vi "ELVIS R meas.vi"(0 "Device Name in":tag="Dev1", 2 "close session":bool, 11 "error in":errorcluster, 12 "Meas type":T1(ring)=enum."Resistance", 13 "Resistance Range (Ohms)":sgl(ring)=100000.0 items=["100ohm"=100, "1Kohm"=1000, "10Kohm"=10000, "100Kohm"=100000, "1Mohm"=1000000, "100Mohm"=1e+08]) -> (4 "Device Name out":tag="Dev1", 8 "Resistance (ohm)":dbl=12101.131778276253, 14 "Overrange":u16(ring) items=["In Range", "+Over", "-Over", "±Over"], 15 "error out":errorcluster)   [LabVIEW 2016]
doc: "Basic Digital Multimeter of NI ELVIS II configured to measure resistance\n\n\nPaul K Dixon\nP350\nCSUSB Physics"
uses:
  <vilib>/express/NI ELVISmx/misc.llb/ctl_ProductType.ctl
  <vilib>/DAQmx/read.llb/DAQmx Read (Analog 1D Wfm NChan NSamp).vi
  <vilib>/DAQmx/read.llb/DAQmx Read (Analog DBL 1Chan 1Samp).vi
  <vilib>/DAQmx/create/channels.llb/DAQmx Create Channel (AI-Voltage-Basic).vi
  <vilib>/DAQmx/create/channels.llb/DAQmx Create Channel (AI-Voltage-RMS).vi
  <vilib>/DAQmx/create/channels.llb/DAQmx Create Channel (AI-Current-Basic).vi
  <vilib>/DAQmx/create/channels.llb/DAQmx Create Channel (AI-Current-RMS).vi
  <vilib>/DAQmx/create/channels.llb/DAQmx Create Channel (AI-Resistance).vi
  <vilib>/DAQmx/create/channels.llb/DAQmx Create Channel (AO-FuncGen).vi
  <vilib>/DAQmx/configure/timing.llb/DAQmx Timing (Sample Clock).vi
  <vilib>/DAQmx/miscellaneous.llb/DAQmx Fill In Error Info.vi
  <vilib>/measure/matone.llb/Extract Single Tone Information 1 Chan.vi
  <resource>/objmgr/daqmx.rc
  <vilib>/measure/NI_MAPro.lvlib
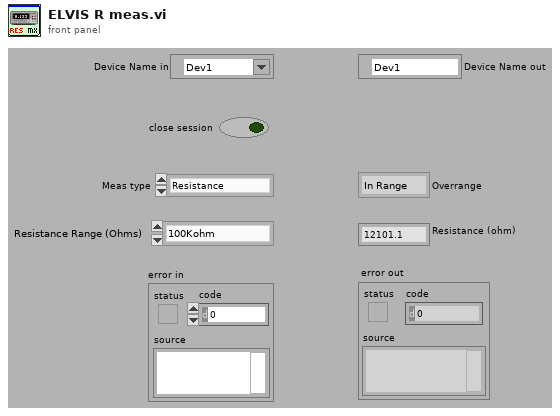
[diagram p1: front panel]
types:
  T1 = enum16{"Volts DC", "Volts AC", "Current DC", "Current AC", "Resistance", "Capacitance", "Inductance", "Diode", "Continuity", "Impedance"}
  T2 = typedef "ctl_ProductType.ctl" = enum16{"NI myDAQ", "NI ELVIS II", "NI ELVIS II+"}
  T3 = cluster{"approx freq. (optional)":dbl, "search (+/- % of Fsampl.)":dbl}
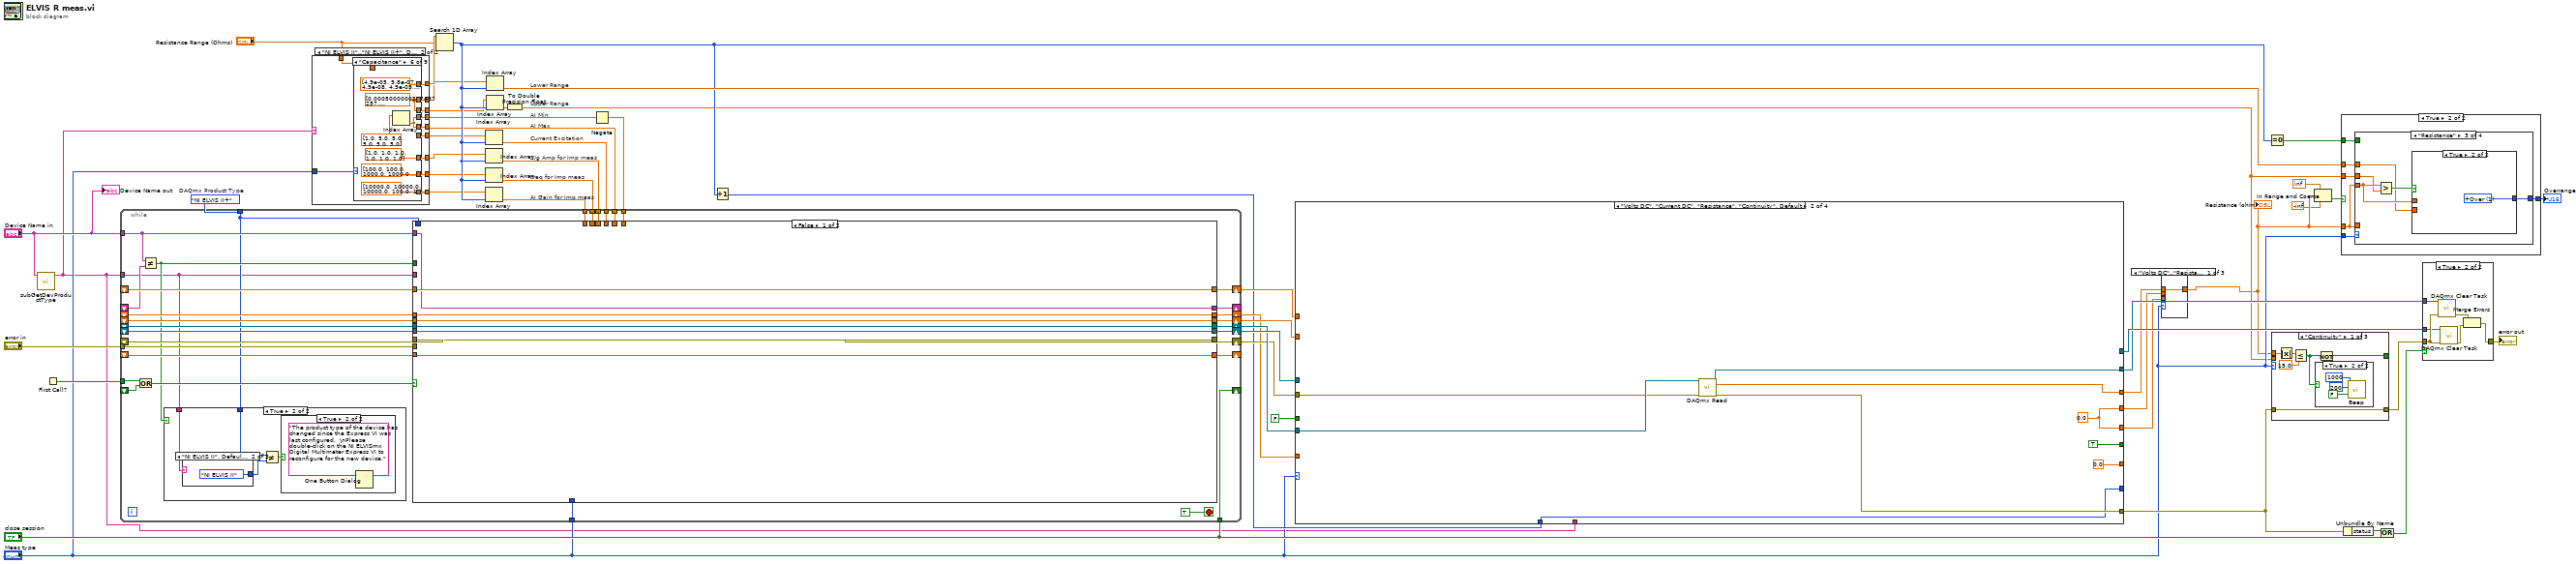
[diagram p0: block diagram]
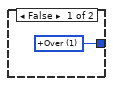
[diagram p2: hidden frame]
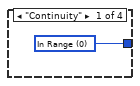
[diagram p3: hidden frame]
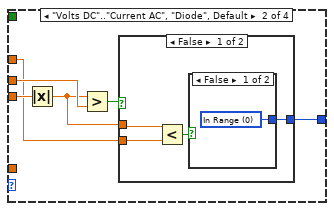
[diagram p4: hidden frame]
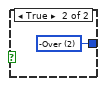
[diagram p5: hidden frame]
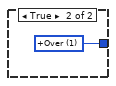
[diagram p6: hidden frame]
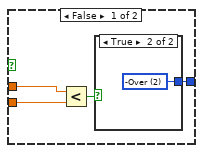
[diagram p7: hidden frame]
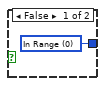
[diagram p8: hidden frame]
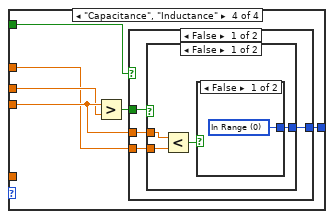
[diagram p9: hidden frame]
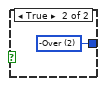
[diagram p10: hidden frame]
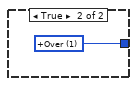
[diagram p11: hidden frame]
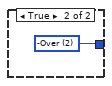
[diagram p12: hidden frame]
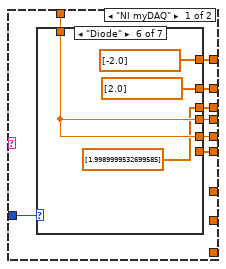
[diagram p13: hidden frame]
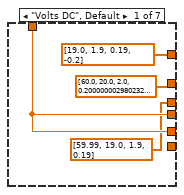
[diagram p14: hidden frame]
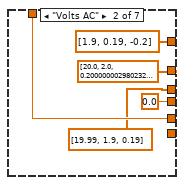
[diagram p15: hidden frame]
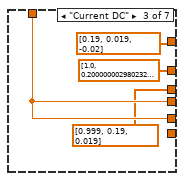
[diagram p16: hidden frame]
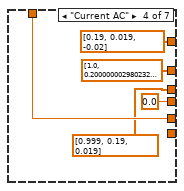
[diagram p17: hidden frame]
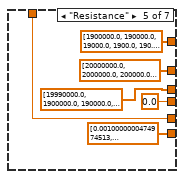
[diagram p18: hidden frame]
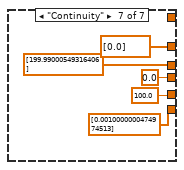
[diagram p19: hidden frame]
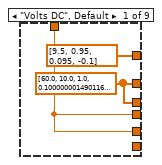
[diagram p20: hidden frame]
diagram:
  w7 = ctl_ProductType."NI ELVIS II+"  # DAQmx Product Type
  # "AI Max"
  # "Lower Range"
  # "Upper Range"
  # "AI Gain for Imp meas"
  # "Freq for Imp meas"
  # "S/g Amp for Imp meas"
  # "AI Min"
  # "Current Excitation"
  n1 = call <vilib>:"subGetDevProductType.vi"("activeDevice"="Device Name in") -> ("DevProductTypeValue"=w5:string)  [unwired: 9 in, 1 out]
  n2 = First Call?() -> (First Call?: T/F=w45:bool)
  n3 = case shown="\"NI ELVIS II\"..\"NI ELVIS II+\", Default" w5 {
    tunnel: [w58 w102] -> w20
    tunnel: [w57 w101] -> w19
    tunnel: [w52 w100] -> w18
    tunnel: [_ w99] -> w17
    tunnel: [_ w98] -> w15
    tunnel: [_ w97] -> w16
    tunnel: "Meas type" -> [w56 w96]
    tunnel: "Resistance Range (Ohms)" -> [w54 w95]
    tunnel: [w55 w94] -> w9
    tunnel: [w53 w93] -> w10
    tunnel: [w51 w92] -> w6
    frame "NI myDAQ" {
      n4 = case shown="\"Diode\"" w56 {
        tunnel: [dbl[] [19.0, 1.9, 0.19, -0.2] dbl[] [1.9, 0.19, -0.2] dbl[] [0.19, 0.019, -0.02] dbl[] [0.19, 0.019, -0.02] dbl[] [1900000.0, 190000.0, 19000.0, 1900.0, 190.0, -1000000000.0] sgl[] [-2.0] _] -> w58
        tunnel: [sgl[] [60.0, 20.0, 2.0, 0.2] sgl[] [20.0, 2.0, 0.2] sgl[] [1.0, 0.2, 0.02] sgl[] [1.0, 0.2, 0.02] sgl[] [20000000.0, 2000000.0, 200000.0, 20000.0, 2000.0, 200.0] sgl[] [2.0] sgl[] [0.0]] -> w57
        tunnel: [w60 sgl 0.0 ("Continuity Input Limits (Ohms)") w69 sgl 0.0 ("Continuity Input Limits (Ohms)") sgl 0.0 ("Continuity Input Limits (Ohms)") w86 sgl 0.0 ("Continuity Input Limits (Ohms)")] -> w55
        tunnel: w54 -> [w60 w64 w69 w73 w79 w86 _]
        tunnel: [w60 w64 w69 w73 w79 w86 sgl 100.0 ("Continuity Input Limits (Ohms)")] -> w53
        tunnel: [_ _ _ _ sgl[] [0.001, 0.001, 0.001, 0.001, 0.001, 0.001] _ sgl[] [0.001]] -> w52
        tunnel: [dbl[] [59.99, 19.0, 1.9, 0.19] dbl[] [19.99, 1.9, 0.19] dbl[] [0.999, 0.19, 0.019] dbl[] [0.999, 0.19, 0.019] dbl[] [19990000.0, 1900000.0, 190000.0, 19000.0, 1900.0, 190.0] dbl[] [1.9989999532699585] dbl[] [199.99000549316406]] -> w51
        frame "Volts DC", Default {
        }
        frame "Volts AC" {
        }
        frame "Current DC" {
        }
        frame "Current AC" {
        }
        frame "Resistance" {
        }
        frame "Diode" {
        }
        frame "Continuity" {
        }
      }
    }
    frame "NI ELVIS II".."NI ELVIS II+", Default {
      n5 = case shown="\"Capacitance\"" w96 {
        tunnel: [dbl[] [9.5, 0.95, 0.095, -0.1] dbl[] [1.9, 0.19, -0.2] dbl[] [0.0] dbl[] [0.48, -0.5] dbl[] [900000.0, 99000.0, 9000.0, 900.0, 90.0, -1000000000.0] dbl[] [4.9e-05, 9.8e-07, 4.9e-08, 4.9e-09, 4.5e-10, inf] dbl[] [0.01, 0.001, 0.0001] dbl[] [0.95, 0.0] _] -> w102
        tunnel: [w103 w106 w110 w113 w117 w122 w129 w136 w139] -> w101
        tunnel: [_ _ _ _ sgl[] [5e-07, 5e-06, 1e-05, 0.0001, 0.001, 0.001] _ _ _ dbl[] [0.001]] -> w100
        tunnel: [_ _ _ _ _ dbl[] [1.0, 1.0, 1.0, 1.0, 1.0, 1.0] dbl[] [1.0, 0.5, 0.5] _ _] -> w99
        tunnel: [_ _ _ _ _ dbl[] [100.0, 100.0, 1000.0, 1000.0, 1000.0, 10000.0] dbl[] [1000.0, 1000.0, 10000.0] _ _] -> w98
        tunnel: [_ _ _ _ _ dbl[] [10000.0, 10000.0, 10000.0, 100.0, 1.0, 1.0] dbl[] [10000.0, 10000.0, 10000.0] _ _] -> w97
        tunnel: w95 -> [w104 w108 w111 w115 w119 _ _ w137 _]
        tunnel: [w104 sgl 0.0 ("Continuity Input Limits (Ohms)") w111 sgl 0.0 ("Continuity Input Limits (Ohms)") sgl 0.0 ("Continuity Input Limits (Ohms)") w123 w130 w137 0.0 ("Continuity Input Limits (Ohms)")] -> w94
        tunnel: [w104 w108 w111 w115 w119 w123 w130 w137 100.0 ("Continuity Input Limits (Ohms)")] -> w93
        tunnel: [w103 w106 w110 w113 w117 w122 w129 w136 w139] -> w92
        frame "Volts DC", Default {
          w103 = sgl[] [60.0, 10.0, 1.0, 0.1]
        }
        frame "Volts AC" {
          w106 = sgl[] [20.0, 2.0, 0.2]
        }
        frame "Current DC" {
          w110 = sgl[] [2.0]
        }
        frame "Current AC" {
          w113 = sgl[] [2.0, 0.5]
        }
        frame "Resistance" {
          w117 = sgl[] [100000000.0, 1000000.0, 100000.0, 10000.0, 1000.0, 100.0]
        }
        frame "Capacitance" {
          w122 = sgl[] [0.0005, 5e-05, 1e-06, 5e-08, 5e-09, 5e-10]
          n6 = Index Array(array=dbl[] [1.0, 5.0, 5.0, 5.0, 5.0, 5.0]) -> (element=w123:dbl)  [unwired: 1 in]
        }
        frame "Inductance" {
          w129 = sgl[] [0.1, 0.01, 0.001]
          n7 = Index Array(array=dbl[] [1.0, 1.0, 1.0]) -> (element=w130:dbl)  [unwired: 1 in]
        }
        frame "Diode" {
          w136 = sgl[] [10.0, 1.0]
        }
        frame "Continuity" {
          w139 = sgl[] [0.0]
        }
      }
    }
  }
  n8 = Search 1D Array(1D array=w19, element="Resistance Range (Ohms)") -> (index of element=w22:i32)  [unwired: 1 in]
  n9 = Index Array(array=w18, index=w22) -> (element=w39:dbl)
  n10 = Index Array(array=w17, index=w22) -> (element=w38:dbl)
  n11 = Index Array(array=w15, index=w22) -> (element=w37:dbl)
  n12 = Index Array(array=w16, index=w22) -> (element=w36:dbl)
  n13 = Index Array(array=w6, index=w22) -> (element=w40:dbl)
  n14 = Index Array(array=w20, index=w22) -> (element=w41:dbl)
  n15 = To Double Precision Float(number=w40) -> (double precision float=w11:dbl)
  n16 = Negate(x=w9) -> (-x=w8:dbl)
  n17 = while {
    tunnel: "error in" -> [w175]
    shift-right: [w174] -> w33
    shift-left: _ -> [w172]
    shift-right: [w170] -> _
    shift-left: _ -> [w169]
    tunnel: "close session" -> [w170]
    tunnel: w45 -> [w167]
    shift-right: [w173] -> w32
    shift-left: _ -> [w166]
    tunnel: "Meas type" -> [w165]
    shift-right: [w164] -> w34
    shift-left: _ -> [w163]
    shift-right: [w162] -> _
    shift-left: _ -> [w146]
    shift-right: [w161] -> w30
    shift-left: _ -> [w160]
    shift-right: [w159] -> _
    shift-left: _ -> [w158]
    shift-right: [w157] -> w31
    shift-left: _ -> [w156]
    shift-right: [w155] -> w35
    shift-left: _ -> [w154]
    tunnel: w5 -> [w143]
    tunnel: w39 -> [w151]
    tunnel: w10 -> [w152]
    tunnel: w38 -> [w150]
    tunnel: w37 -> [w149]
    tunnel: w36 -> [w153]
    tunnel: "Device Name in" -> [w147]
    tunnel: w8 -> [w148]
    tunnel: w7 -> [w144]
    stop <- TRUE stop-if-true
    n18 = Or(x=w167, y=w169) -> (x .or. y?=w168:bool)
    n19 = Not Equal?(x=w147, y=w146) -> (x != y?=w145:bool)
    n20 = case shown="True" w145 {
      tunnel: w144 -> [_ w178]
      tunnel: w143 -> [_ w176]
      frame False {
      }
      frame True {
        n21 = case shown="\"NI ELVIS II\", Default" w176 {
          tunnel: [ctl_ProductType."NI ELVIS II+" ("Product Type") ctl_ProductType."NI ELVIS II" ("Product Type") ctl_ProductType."NI myDAQ" ("Product Type")] -> w179
          frame "NI ELVIS II+" {
          }
          frame "NI ELVIS II", Default {
          }
          frame "NI myDAQ" {
          }
        }
        n22 = Not Equal?(x=w178, y=w179) -> (x != y?=w177:bool)
        n23 = case shown="True" w177 {
          frame False {
          }
          frame True {
            n24 = One Button Dialog(message="The product type of the device has changed since the Express VI was last configured.  \nPlease double-click on the NI ELVISmx Digital Multimeter Express VI to reconfigure for the new device.") -> ()  [unwired: 1 in, 1 out]
          }
        }
      }
    }
    n25 = case shown="False" w168 {
      tunnel: w175 -> [_ w213]
      tunnel: [w191 w199] -> w174
      tunnel: [w190 w197] -> w173
      tunnel: w172 -> [w191 _]
      tunnel: w166 -> [w190 _]
      tunnel: w165 -> [_ w206]
      tunnel: [w189 w198] -> w164
      tunnel: w163 -> [w189 _]
      tunnel: [w184 w195] -> w162
      tunnel: [w188 w196] -> w161
      tunnel: w160 -> [w188 _]
      tunnel: [w186 w205] -> w159
      tunnel: w158 -> [w186 w210]
      tunnel: [w187 w201] -> w157
      tunnel: w156 -> [w187 _]
      tunnel: [w185 w200] -> w155
      tunnel: w154 -> [w185 _]
      tunnel: w143 -> [_ w193]
      tunnel: w153 -> [_ w196]
      tunnel: w152 -> [_ w209]
      tunnel: w151 -> [_ w208]
      tunnel: w150 -> [_ w207]
      tunnel: w149 -> [_ w200]
      tunnel: w147 -> [w184 w195]
      tunnel: w148 -> [_ w194]
      tunnel: w144 -> [_ _]
      tunnel: w145 -> [_ w192]
      frame False {
      }
      frame True {
        n26 = First Call?() -> (First Call?: T/F=w212:bool)
        n27 = Or(x=w192, y=w212) -> (x .or. y?=w211:bool)
        n28 = case shown="\"NI ELVIS II\", Default" w193 {
          tunnel: w213 -> [w333 w339]
          tunnel: [w333 w338] -> w204
          tunnel: w211 -> [_ w337]
          tunnel: w195 -> [_ w336]
          tunnel: [w332 w335] -> w205
          tunnel: w210 -> [w332 w334]
          frame "NI myDAQ" {
          }
          frame "NI ELVIS II", Default {
            n29 = case shown="True" w337 {
              tunnel: w339 -> [w341 w345]
              tunnel: [w341 w344] -> w338
              tunnel: w336 -> [_ w343]
              tunnel: [w340 w342] -> w335
              tunnel: w334 -> [w340 _]
              frame False {
              }
              frame True {
                n30 = call <vilib>:"subRecordEEPROMValues.vi"("error in"=w345, "Device Name"=w343) -> ("error out"=w344:errorcluster, "Resistance Array"=w342:sgl[])  [unwired: 8 in]
              }
            }
          }
        }
        n31 = call <vilib>:"DAQmx Create Task.vi"("error in"=w204) -> ("task out"=w202:refnum<k21>, "error out"=w203:errorcluster)  [unwired: 13 in]
        n32 = case shown="\"Volts AC\"" w206 {
          tunnel: w195 -> [w222 w231 w240 w249 w262 w280 w290]
          tunnel: w202 -> [w219 w228 w237 w246 w259 w277 _]
          tunnel: w203 -> [w218 w227 w236 w245 w258 w276 w288]
          tunnel: [w217 w226 w235 w244 w257 w273 w285] -> w199
          tunnel: [_ _ _ _ _ _ w286] -> w198
          tunnel: [w216 w225 w234 w243 w256 w274 w284] -> w197
          tunnel: w194 -> [w215 w224 w233 w242 w252 w271 w282]
          tunnel: w209 -> [w214 w223 w232 w241 w251 w270 w293]
          tunnel: w208 -> [_ _ _ _ w250 _ _]
          tunnel: [_ _ _ _ _ _ w287] -> w201
          tunnel: w205 -> [_ _ _ _ _ _ w289]
          tunnel: w200 -> [_ _ _ _ _ _ w283]
          tunnel: w207 -> [_ _ _ _ _ _ w291]
          tunnel: w196 -> [_ _ _ _ _ _ w292]
          frame "Volts DC", Default {
            n33 = Format Into String(format string="%s/dmm", w222) -> (resulting string=w220:string)  [unwired: 2 in, 1 out]
            n34 = call-poly <vilib>:"DAQmx Create Virtual Channel.vi"("task in"=w219, "maximum value"=w214, "minimum value"=w215, "physical channels"=w220, "error in"=w218) -> ("task out"=w217:refnum<k21>, "error out"=w216:errorcluster)  [unwired: 9 in]
          }
          frame "Volts AC" {
            n35 = Format Into String(format string="%s/dmm", w231) -> (resulting string=w229:string)  [unwired: 2 in, 1 out]
            n36 = call-poly <vilib>:"DAQmx Create Virtual Channel.vi"("task in"=w228, "maximum value"=w223, "minimum value"=w224, "physical channels"=w229, "error in"=w227) -> ("task out"=w226:refnum<k21>, "error out"=w225:errorcluster)  [unwired: 9 in]
          }
          frame "Current DC" {
            n37 = Format Into String(format string="%s/dmm", w240) -> (resulting string=w238:string)  [unwired: 2 in, 1 out]
            n38 = call-poly <vilib>:"DAQmx Create Virtual Channel.vi"("task in"=w237, "maximum value"=w232, "minimum value"=w233, "physical channels"=w238, "error in"=w236) -> ("task out"=w235:refnum<k21>, "error out"=w234:errorcluster)  [unwired: 9 in]
          }
          frame "Current AC" {
            n39 = Format Into String(format string="%s/dmm", w249) -> (resulting string=w247:string)  [unwired: 2 in, 1 out]
            n40 = call-poly <vilib>:"DAQmx Create Virtual Channel.vi"("task in"=w246, "maximum value"=w241, "minimum value"=w242, "physical channels"=w247, "error in"=w245) -> ("task out"=w244:refnum<k21>, "error out"=w243:errorcluster)  [unwired: 9 in]
          }
          frame "Resistance", "Continuity" {
            w253 = 2 items=["2-Wire"=2, "3-Wire"=3, "4-Wire"=4] ("resistance configuration")
            w254 = 10384 items=["Ohms"=10384, "From Custom Scale"=10065] ("units")
            w255 = 10200 items=["Internal"=10200, "External"=10167, "None"=10230] ("current excitation source")
            n41 = Format Into String(format string="%s/dmm", w262) -> (resulting string=w260:string)  [unwired: 2 in, 1 out]
            n42 = call-poly <vilib>:"DAQmx Create Virtual Channel.vi"("task in"=w259, "maximum value"=w251, "minimum value"=w252, "resistance configuration"=w253, "physical channels"=w260, "units"=w254, "current excitation value"=w250, "error in"=w258, "current excitation source"=w255) -> ("task out"=w257:refnum<k21>, "error out"=w256:errorcluster)  [unwired: 5 in]
          }
          frame "Diode" {
            w272 = 10200 items=["Internal"=10200, "External"=10167, "None"=10230] ("AI.Excit.Src")
            n43 = Format Into String(format string="%s/dmm", w280) -> (resulting string=w275:string)  [unwired: 2 in, 1 out]
            n44 = call-poly <vilib>:"DAQmx Create Virtual Channel.vi"("task in"=w277, "maximum value"=w270, "minimum value"=w271, "physical channels"=w275, "error in"=w276) -> ("task out"=w278:refnum<k21>, "error out"=w279:errorcluster)  [unwired: 9 in]
            n45 = Equal?(x=w270, y=10.0) -> (x = y?=w268:bool)
            n46 = Select(t=0.0001, s=w268, f=0.001) -> (s? t:f=w265:dbl)
            n47 = property class="DAQmx Channel"(reference=w278, error in=w279, "AI.Excit.Src"=w272, "AI.Excit.Val"=w265) -> (reference out=w263:refnum<k21>, error out=w264:errorcluster)
            n48 = call <vilib>:"DAQmx Start Task.vi"("task/channels in"=w263, "error in"=w264) -> ("task out"=w273:refnum<k21>, "error out"=w274:errorcluster)  [unwired: 12 in]
          }
          frame "Capacitance", "Inductance" {
            w300 = 10178 items=["Finite Samples"=10178, "Continuous Samples"=10123, "Hardware Timed Single Point"=12522] ("sample mode")
            w294 = 14751 items=["Sine"=14751, "Triangle"=14752, "Square"=14753, "Sawtooth"=14754] ("type")
            n49 = Format Into String(format string="%s/_DUTPos", w290) -> (resulting string=w304:string)  [unwired: 2 in, 1 out]
            n50 = Format Into String(format string="%s/_DUTNeg", w290) -> (resulting string=w303:string)  [unwired: 2 in, 1 out]
            n51 = Format Into String(format string="%s/_fgenImpedance", w290) -> (resulting string=w295:string)  [unwired: 2 in, 1 out]
            n52 = call <vilib>:"DAQmx Create Task.vi"("error in"=w288) -> ("task out"=w297:refnum<k21>, "error out"=w296:errorcluster)  [unwired: 13 in]
            n53 = Build Array(w304, w303) -> (w302:string[])
            n54 = call-poly <vilib>:"DAQmx Create Virtual Channel.vi"("task in"=w297, "frequency"=w283, "amplitude"=w291, "physical channels"=w295, "type"=w294, "error in"=w296) -> ("task out"=w286:refnum<k21>, "error out"=w312:errorcluster)  [unwired: 8 in]
            n55 = case shown="10000, Default" w292 {
              tunnel: [2 ("index") 1 ("index") 0 ("index")] -> w311
              frame 10000, Default {
              }
              frame 100 {
              }
              frame 1 {
              }
            }
            n56 = call <vilib>:"DAQmx Create Task.vi"("error in"=w312) -> ("task out"=w301:refnum<k21>, "error out"=w299:errorcluster)  [unwired: 13 in]
            n57 = Index Array(array=w289, index=w311) -> (element=w287:sgl)
            n58 = for {
              tunnel: w302 -> [w328] mode=indexing
              shift-right: [w326] -> w308
              shift-left: w299 -> [w329]
              shift-right: [w327] -> w310
              shift-left: w301 -> [w330]
              tunnel: w293 -> [w325]
              tunnel: w282 -> [w324]
              w331 = 10083 items=["default"=-1, "RSE"=10083, "NRSE"=10078, "Differential"=10106, "Pseudodifferential"=12529] ("input terminal configuration")
              n59 = call-poly <vilib>:"DAQmx Create Virtual Channel.vi"("task in"=w330, "maximum value"=w325, "minimum value"=w324, "input terminal configuration"=w331, "physical channels"=w328, "error in"=w329) -> ("task out"=w327:refnum<k21>, "error out"=w326:errorcluster)  [unwired: 8 in]
            }
            n60 = property class="DAQmx Channel"(reference=w310, error in=w308, "AI.Gain"=w292) -> (reference out=w307:refnum<k21>, error out=w309:errorcluster)
            n61 = Greater?(x=w283, y=200.0) -> (0:w314:bool)
            n62 = case shown="False" w314 {
              tunnel: [25000 ("samples per channel") 250000 ("samples per channel")] -> w316
              tunnel: [50000.0 ("rate") 500000.0 ("rate")] -> w315
              frame False {
              }
              frame True {
              }
            }
            n63 = call-poly <vilib>:"DAQmx Timing.vi"("task/channels in"=w307, "sample mode"=w300, "samples per channel"=w316, "rate"=w315, "error in"=w309) -> ("task out"=w285:refnum<k21>, "error out"=w284:errorcluster)  [unwired: 9 in]
          }
        }
      }
    }
  }
  n64 = Increment(x=w22) -> (x+1=w21:i32)
  n65 = case shown="\"Volts DC\", \"Current DC\", \"Resistance\", \"Continuity\", Default" "Meas type" {
    selector: "Meas type" -> [w358 _ _ _]
    tunnel: w34 -> [w403 _ _ _]
    tunnel: w32 -> [w402 w475 w489 w540]
    tunnel: w33 -> [w392 w476 w490 w541]
    tunnel: w30 -> [w391 _ _ _]
    tunnel: [w401 _ _ _] -> w28
    tunnel: [w400 w473 w484 w534] -> w27
    tunnel: [w346 w472 w482 w536] -> w23
    tunnel: [0.0 ("data") w474 w483 w535] -> w26
    tunnel: [w349 w477 w491 w542] -> w25
    tunnel: [w350 w477 w491 w542] -> w24
    tunnel: w31 -> [w354 _ _ _]
    tunnel: [w351 0.0 ("Computed Value") 0.0 ("Computed Value") 0.0 ("Computed Value")] -> _
    tunnel: FALSE ("Run Once?") -> [w353 _ w485 _]
    tunnel: [w347 w470 w487 w538] -> _
    tunnel: w21 -> [w352 w470 w487 w538]
    tunnel: [w348 TRUE ("Good Range?") TRUE ("Good Range?") TRUE ("Good Range?")] -> _
    tunnel: w35 -> [w355 _ _ _]
    tunnel: w5 -> [_ _ w478 _]
    frame "Capacitance", "Inductance" {
      n66 = call <vilib>:"DAQmx Start Task.vi"("task/channels in"=w403, "error in"=w402) -> ("task out"=w397:refnum<k21>, "error out"=w398:errorcluster)  [unwired: 12 in]
      n67 = call <vilib>:"DAQmx Stop Task.vi"("task/channels in"=w397, "error in"=w398) -> ("task out"=w401:refnum<k21>, "error out"=w394:errorcluster)  [unwired: 12 in]
      n68 = property class="DAQmx Channel"(reference=w392, error in=w394, "AI.Gain"=w391) -> (reference out=w395:refnum<k21>, error out=w393:errorcluster)
      n69 = call-poly <vilib>:"DAQmx Read.vi"("task/channels in"=w395, "error in"=w393) -> ("task out"=w400:refnum<k21>, "data"=w396:waveform(dbl)[], "error out"=w346:errorcluster)  [unwired: 11 in]
      n70 = Index Array(array=w396) -> (element #1=w357:waveform(dbl), element #2=w390:waveform(dbl))  [unwired: 2 in]
      n71 = Negate(x=w390) -> (-x=w356:waveform(dbl))
      n72 = Bundle By Name(cluster=T3 {"approx freq. (optional)"=-1.0, "search (+/- % of Fsampl.)"=5.0} ("advanced search"), "approx freq. (optional)"=w355, "search (+/- % of Fsampl.)"=1.0) -> (w359:T3)
      n73 = call-poly <vilib>:"Extract Single Tone Information.vi"("advanced search"=w359, "time signal in"=w357) -> ("detected phase (deg)"=w383:dbl, "detected amplitude"=w385:dbl, "detected frequency"=w387:dbl)  [unwired: 4 in, 3 out]
      n74 = call-poly <vilib>:"Extract Single Tone Information.vi"("advanced search"=w359, "time signal in"=w356) -> ("detected phase (deg)"=w382:dbl, "detected amplitude"=w389:dbl)  [unwired: 4 in, 4 out]
      n75 = Divide(x=w389, y=w354) -> (x/y=w386:dbl)
      n76 = Divide(x=w385, y=w386) -> (x/y=w384:dbl)
      n77 = Subtract(x=w383, y=w382) -> (x-y=w365:dbl)
      n78 = case shown="True" w353 {
        tunnel: w352 -> [w405 w409]
        tunnel: w389 -> [_ w410]
        tunnel: [w405 w408] -> w347
        tunnel: [TRUE w407] -> w348
        tunnel: w358 -> [_ w406]
        frame False {
        }
        frame True {
          n79 = Greater?(x=w410, y=4.2) -> (0:w411:bool)
          n80 = case shown="True" w411 {
            tunnel: w410 -> [w419 _]
            tunnel: w409 -> [w416 w439]
            tunnel: [w415 w440] -> w408
            tunnel: [w414 FALSE] -> w407
            tunnel: w406 -> [w413 _]
            frame False {
              n81 = Less?(x=w419, y=0.001) -> (x < y?=w417:bool)
              n82 = case shown="True" w417 {
                tunnel: w416 -> [w421 w424]
                tunnel: [w421 w423] -> w415
                tunnel: [TRUE FALSE] -> w414
                tunnel: w413 -> [_ w422]
                frame False {
                }
                frame True {
                  n83 = case shown="Default" w422 {
                    tunnel: w424 -> [w427 w431 w436]
                    tunnel: [w426 w431 w434] -> w423
                    frame "Inductance" {
                      w428 = 3 ("y")
                      n84 = Equal?(x=w428, y=w427) -> (x = y?=w430:bool)
                      n85 = Increment(x=w427) -> (x+1=w429:i32)
                      n86 = Select(t=w428, s=w430, f=w429) -> (s? t:f=w426:i32)
                    }
                    frame Default {
                    }
                    frame "Capacitance" {
                      w432 = 6 ("y")
                      n87 = Equal?(x=w432, y=w436) -> (x = y?=w435:bool)
                      n88 = Increment(x=w436) -> (x+1=w433:i32)
                      n89 = Select(t=w432, s=w435, f=w433) -> (s? t:f=w434:i32)
                    }
                  }
                }
              }
            }
            frame True {
              w437 = 1 ("x")
              n90 = Equal?(x=w437, y=w439) -> (x = y?=w441:bool)
              n91 = Decrement(x=w439) -> (x-1=w438:i32)
              n92 = Select(t=w437, s=w441, f=w438) -> (s? t:f=w440:i32)
            }
          }
        }
      }
      n93 = Subtract(x=w365, y=360.0) -> (x-y=w378:dbl)
      n94 = Greater?(x=w365, y=180.0) -> (0:w380:bool)
      n95 = Select(t=w378, s=w380, f=w365) -> (s? t:f=w373:dbl)
      n96 = Add(x=w365, y=360.0) -> (x+y=w374:dbl)
      n97 = Less?(x=w373, y=-180.0) -> (x < y?=w376:bool)
      n98 = Select(t=w374, s=w376, f=w373) -> (s? t:f=w364:dbl)
      n99 = In Range and Coerce(upper limit=90.0, x=w364, lower limit=-90.0) -> (coerced(x)=w363:dbl)  [unwired: 1 out]
      n100 = Divide(x=3.141592653589793 ("Pi"), y=180.0) -> (x/y=w370:dbl)
      n101 = Multiply(x=w363, y=w370) -> (x*y=w369:dbl)
      n102 = Sine(x=w369) -> (sin(x)=w368:dbl)
      n103 = Multiply(x=w384, y=w368) -> (x*y=w388:dbl)
      n104 = Less Than 0?(x=w388) -> (x < 0?=w362:bool)
      n105 = case shown="\"Capacitance\"" w358 {
        tunnel: w387 -> [w445 _ w450]
        tunnel: w388 -> [w444 _ w449]
        tunnel: [w443 _ w448] -> w351
        frame "Inductance" {
          n106 = Multiply(x=6.283185307179586 ("Pi Multiplied By 2"), y=w445) -> (x*y=w447:dbl)
          n107 = Divide(x=w444, y=w447) -> (x/y=w443:dbl)
        }
        frame Default {
        }
        frame "Capacitance" {
          n108 = Multiply(x=6.283185307179586 ("Pi Multiplied By 2"), y=w450) -> (x*y=w453:dbl)
          n109 = Negate(x=w449) -> (-x=w452:dbl)
          n110 = Multiply(x=w453, y=w452) -> (x*y=w454:dbl)
          n111 = Reciprocal(x=w454) -> (1/x=w448:dbl)
        }
      }
      n112 = case shown="True" w362 {
        tunnel: w387 -> [w458 w467]
        tunnel: w388 -> [w457 w463]
        tunnel: [w456 inf ("Positive Infinity")] -> w349
        tunnel: [inf ("Positive Infinity") w466] -> w350
        frame True {
          n113 = Multiply(x=6.283185307179586 ("Pi Multiplied By 2"), y=w458) -> (x*y=w461:dbl)
          n114 = Negate(x=w457) -> (-x=w460:dbl)
          n115 = Multiply(x=w461, y=w460) -> (x*y=w462:dbl)
          n116 = Reciprocal(x=w462) -> (1/x=w456:dbl)
        }
        frame False {
          n117 = Multiply(x=6.283185307179586 ("Pi Multiplied By 2"), y=w467) -> (x*y=w464:dbl)
          n118 = Divide(x=w463, y=w464) -> (x/y=w466:dbl)
        }
      }
    }
    frame "Volts DC", "Current DC", "Resistance", "Continuity", Default {
      w477 = 0.0 ("Phase")
      n119 = call-poly <vilib>:"DAQmx Read.vi"("task/channels in"=w476, "error in"=w475) -> ("task out"=w473:refnum<k21>, "data"=w474:dbl, "error out"=w472:errorcluster)  [unwired: 11 in]
    }
    frame "Volts AC", "Current AC" {
      w491 = 0.0 ("Phase")
      n120 = call-poly <vilib>:"DAQmx Read.vi"("task/channels in"=w490, "error in"=w489) -> ("task out"=w481:refnum<k21>, "data"=w480:dbl, "error out"=w479:errorcluster)  [unwired: 11 in]
      n121 = case shown="\"NI ELVIS II\", Default" w478 {
        tunnel: w485 -> [_ w503]
        tunnel: [w493 w502] -> w484
        tunnel: [w494 w501] -> w483
        tunnel: [w492 w500] -> w482
        tunnel: w481 -> [w493 w499]
        tunnel: w480 -> [w494 w498]
        tunnel: w479 -> [w492 w497]
        frame "NI myDAQ" {
          # "No need to add the delay or to discard the initial readings for myDAQ."
        }
        frame "NI ELVIS II", Default {
          # "This is a workaround for the issue with ELVIS II/II+ AC measurements"
          n122 = Build Array(w503, TRUE ("Run Once?")) -> (w504:bool[])
          n123 = Boolean Array To Number(Boolean array=w504) -> (number=w496:u32)
          n124 = case shown="2" w496 {
            tunnel: w498 -> [w506 _ _]
            tunnel: w499 -> [w505 w513 w525]
            tunnel: w497 -> [w507 w512 w522]
            tunnel: [w507 w511 w521] -> w500
            tunnel: [w506 w510 w523] -> w501
            tunnel: [w505 w509 w524] -> w502
            frame 0, Default {
              # "Specific Range, Run Continuous"
            }
            frame 1, 3 {
              # "Auto Range, Run Continuous/Run Once"
              n125 = for {
                N: 3 -> [_]
                tunnel: w513 -> [w518]
                tunnel: w512 -> [w517]
                tunnel: [w516] -> w511
                tunnel: [w515] -> w510
                tunnel: [w514] -> w509
                n126 = call-poly <vilib>:"DAQmx Read.vi"("task/channels in"=w518, "error in"=w517) -> ("task out"=w514:refnum<k21>, "data"=w515:dbl, "error out"=w516:errorcluster)  [unwired: 11 in]
              }
            }
            frame 2 {
              # "Specific Range, Run Once"
              n127 = flat-sequence {
                tunnel: w522 -> [w527]
                tunnel: w525 -> [w528]
                tunnel: [w528] -> w520
                tunnel: [w527] -> w519
                tunnel: [w531] -> w524
                tunnel: [w529] -> w523
                tunnel: [w530] -> w521
                tunnel: w520 -> [w533]
                tunnel: w519 -> [w532]
                tunnel: [w529] -> _
                frame #0 {
                  n128 = Wait Until Next ms Multiple(millisecond multiple=u32 5000) -> ()  [unwired: 1 out]
                }
                frame #1 {
                  n129 = call-poly <vilib>:"DAQmx Read.vi"("task/channels in"=w533, "error in"=w532) -> ("task out"=w531:refnum<k21>, "data"=w529:dbl, "error out"=w530:errorcluster)  [unwired: 11 in]
                }
              }
            }
          }
        }
      }
    }
    frame "Diode" {
      w542 = 0.0 ("Phase")
      n130 = call-poly <vilib>:"DAQmx Read.vi"("task/channels in"=w541, "error in"=w540) -> ("task out"=w534:refnum<k21>, "data"=w535:dbl, "error out"=w536:errorcluster)  [unwired: 11 in]
    }
  }
  n131 = case shown="\"Volts DC\"..\"Resistance\", \"Diode\", \"Continuity\", Default" "Meas type" {
    tunnel: w26 -> [w543 _ _]
    tunnel: w25 -> [_ w544 _]
    tunnel: w24 -> [_ _ w545]
    tunnel: [w543 w544 w545] -> w4
    frame "Volts DC".."Resistance", "Diode", "Continuity", Default {
    }
    frame "Capacitance" {
    }
    frame "Inductance" {
    }
  }
  "Resistance (ohm)" <- w4
  n132 = Equal To 0?(x=w22) -> (x = 0?=w42:bool)
  n133 = case shown="\"Continuity\"" "Meas type" {
    tunnel: w4 -> [w551 _ w560]
    tunnel: w23 -> [w550 w555 w559]
    tunnel: [w550 w555 w559] -> w44
    tunnel: [w546 _ w557] -> _
    tunnel: w11 -> [_ _ w556]
    frame "Continuity" {
      n134 = Absolute Value(x=w551) -> (abs(x)=w548:dbl)
      n135 = Less Or Equal?(x=w548, y=15.0) -> (x <= y?=w547:bool)
      n136 = case shown="True" w547 {
        frame False {
        }
        frame True {
          n137 = call <vilib>:"Beep.vi"("use system alert? (T)"=FALSE, "duration (msec)"=u32 200, "frequency (Hz)"=u32 1000) -> ()  [unwired: 9 in]
        }
      }
      n138 = Not(x=w547) -> (.not. x?=w546:bool)
    }
    frame Default {
    }
    frame "Diode" {
      n139 = Less Or Equal?(x=w560, y=w556) -> (x <= y?=w558:bool)
      n140 = Not(x=w558) -> (.not. x?=w557:bool)
    }
  }
  n141 = In Range and Coerce(upper limit=inf ("Positive Infinity"), x=w4, lower limit=-inf ("Negative Infinity")) -> (In Range?=w1:bool)  [unwired: 1 out]
  n142 = case shown="True" w1 {
    tunnel: w4 -> [_ w567]
    tunnel: [w561 w566] -> w43
    tunnel: w42 -> [_ w565]
    tunnel: w41 -> [_ w564]
    tunnel: "Meas type" -> [_ w563]
    tunnel: w11 -> [_ w562]
    frame False {
      w561 = u16 1 items=["In Range", "+Over", "-Over", "±Over"] ("Overrange")
    }
    frame True {
      n143 = case shown="\"Resistance\"" w563 {
        tunnel: w567 -> [_ _ _ _]
        tunnel: w567 -> [_ w571 w584 w597]
        tunnel: [w568 w573 w585 w598] -> w566
        tunnel: w562 -> [_ w572 w583 w596]
        tunnel: w564 -> [_ w569 w582 w595]
        tunnel: w565 -> [_ _ _ w594]
        frame "Continuity" {
          w568 = u16 0 items=["In Range", "+Over", "-Over", "±Over"] ("Overrange")
        }
        frame "Volts DC".."Current AC", "Diode", Default {
          n144 = Absolute Value(x=w571) -> (abs(x)=w570:dbl)
          n145 = Greater?(x=w570, y=w572) -> (0:w574:bool)
          n146 = case shown="False" w574 {
            tunnel: w569 -> [w578 _]
            tunnel: w570 -> [w577 _]
            tunnel: [w575 w581] -> w573
            frame False {
              n147 = Less?(x=w577, y=w578) -> (x < y?=w576:bool)
              n148 = case shown="False" w576 {
                tunnel: [w579 w580] -> w575
                frame False {
                  w579 = u16 0 items=["In Range", "+Over", "-Over", "±Over"] ("Overrange")
                }
                frame True {
                  w580 = u16 2 items=["In Range", "+Over", "-Over", "±Over"] ("Overrange")
                }
              }
            }
            frame True {
              w581 = u16 1 items=["In Range", "+Over", "-Over", "±Over"] ("Overrange")
            }
          }
        }
        frame "Resistance" {
          n149 = Greater?(x=w584, y=w583) -> (0:w586:bool)
          n150 = case shown="True" w586 {
            tunnel: w582 -> [w590 _]
            tunnel: w584 -> [w589 _]
            tunnel: [w587 w593] -> w585
            frame False {
              n151 = Less?(x=w589, y=w590) -> (x < y?=w588:bool)
              n152 = case shown="True" w588 {
                tunnel: [w591 w592] -> w587
                frame False {
                  w591 = u16 0 items=["In Range", "+Over", "-Over", "±Over"] ("Overrange")
                }
                frame True {
                  w592 = u16 2 items=["In Range", "+Over", "-Over", "±Over"] ("Overrange")
                }
              }
            }
            frame True {
              w593 = u16 1 items=["In Range", "+Over", "-Over", "±Over"] ("Overrange")
            }
          }
        }
        frame "Capacitance", "Inductance" {
          n153 = Greater?(x=w597, y=w596) -> (0:w599:bool)
          n154 = case shown="False" w594 {
            tunnel: w599 -> [w603 _]
            tunnel: [w602 w611] -> w598
            tunnel: w597 -> [w601 _]
            tunnel: w595 -> [w600 _]
            frame False {
              n155 = case shown="False" w603 {
                tunnel: w600 -> [w607 _]
                tunnel: w601 -> [w606 _]
                tunnel: [w604 w610] -> w602
                frame False {
                  n156 = Less?(x=w606, y=w607) -> (x < y?=w605:bool)
                  n157 = case shown="False" w605 {
                    tunnel: [w608 w609] -> w604
                    frame False {
                      w608 = u16 0 items=["In Range", "+Over", "-Over", "±Over"] ("Overrange")
                    }
                    frame True {
                      w609 = u16 2 items=["In Range", "+Over", "-Over", "±Over"] ("Overrange")
                    }
                  }
                }
                frame True {
                  w610 = u16 1 items=["In Range", "+Over", "-Over", "±Over"] ("Overrange")
                }
              }
            }
            frame True {
              w611 = u16 2 items=["In Range", "+Over", "-Over", "±Over"] ("Overrange")
            }
          }
        }
      }
    }
  }
  "Overrange" <- w43
  n158 = Unbundle By Name(w23) -> ("status"=w48:bool)
  n159 = Or(x=w48, y="close session") -> (x .or. y?=w47:bool)
  n160 = case shown="True" w47 {
    tunnel: [w612 w616] -> w49
    tunnel: w44 -> [w612 w615]
    tunnel: w27 -> [_ w614]
    tunnel: w28 -> [_ w613]
    frame False {
    }
    frame True {
      n161 = call <vilib>:"DAQmx Clear Task.vi"("task in"=w614, "error in"=w615) -> ("error out"=w618:errorcluster)  [unwired: 13 in]
      n162 = call <vilib>:"DAQmx Clear Task.vi"("task in"=w613, "error in"=w615) -> ("error out"=w617:errorcluster)  [unwired: 13 in]
      n163 = Merge Errors(w618, w617) -> (w616:errorcluster)
    }
  }
  "error out" <- w49
  "Device Name out" <- "Device Name in"
